vi "设备编号.vi"() -> ()   [LabVIEW 2013]
panel:
  in  "设备编号":u8
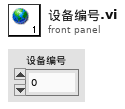
[diagram p1: front panel]
diagram:
